vi "img test6.vi"() -> ()   [LabVIEW 2009]
uses:
  <vilib>/vision/NI_Vision_Development_Module.lvlib
panel:
  in  "start":i32
  out "Image 5":T1(plugin-control)
  out "Image 3":T1(plugin-control)
  in  "Range":cluster{"Lower value":sgl, "Upper value":sgl}={"Lower value"=30.0, "Upper value"=90.0} {"Upper value" format="%.2f"; "Lower value" format="%.2f"}
  out "Image 2":T1(plugin-control)
  in  "AVI Path":path=path "C:/Users/Kokum Weeratunga/Desktop/img processing/ChongWei vs LinDan (japan open 2010).avi"
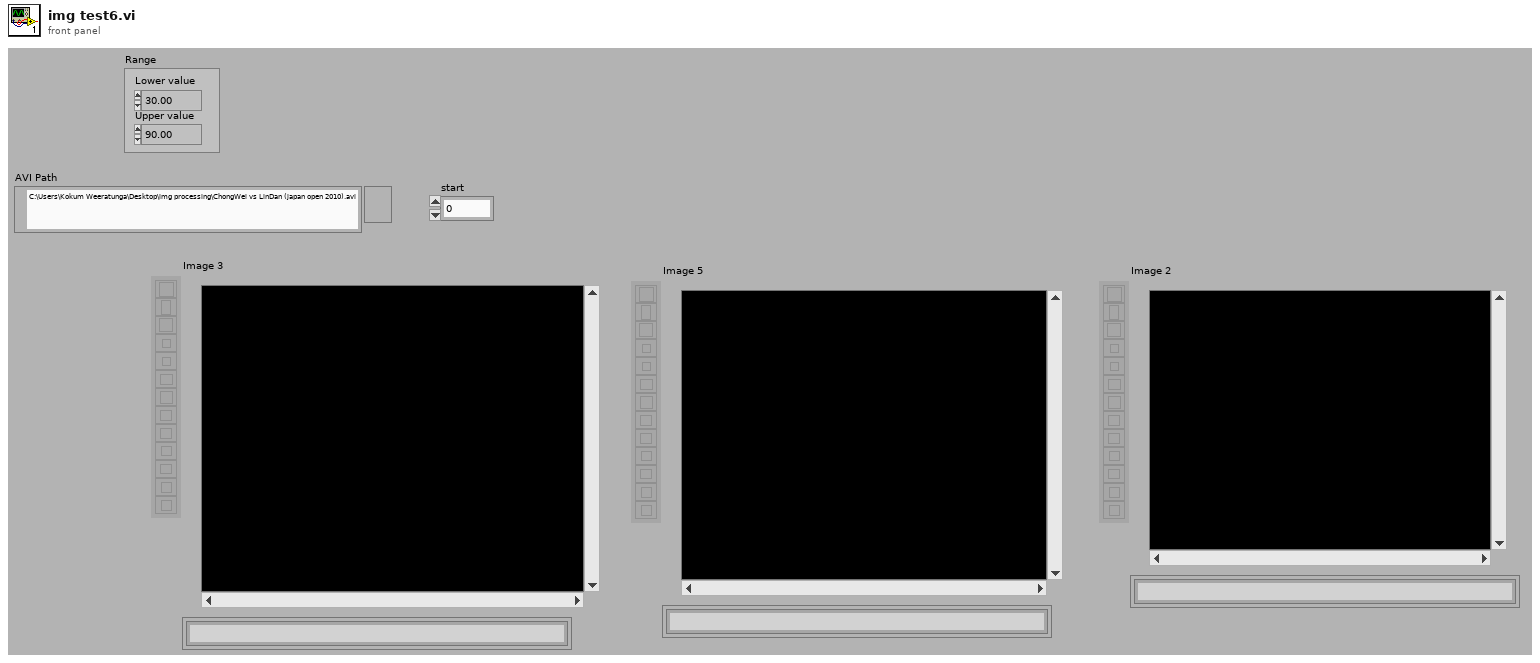
[diagram p1: front panel]
types:
  T1 = typedef "IMAQ Image.ctl" = refnum<image>
  T2 = typedef "Image Type" = u32
  T3 = typedef "AviRefnum.ctl" = refnum<k1>
  T4 = enum32{"AutoM", "Close", "Dilate", "Erode", "Gradient", "Gradient in", "Gradient out", "HitMiss", "Open", "PClose", "POpen", "Thick", "Thin"}
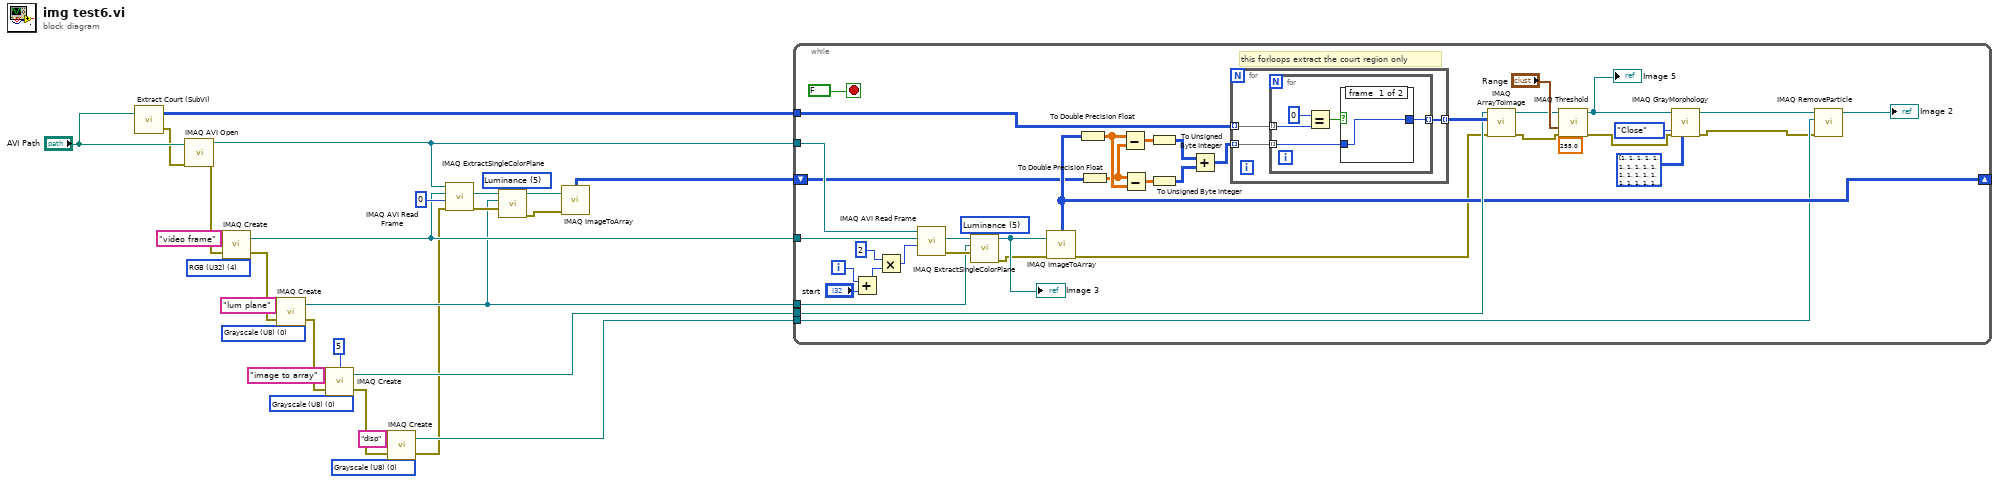
[diagram p0: block diagram]
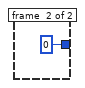
[diagram p2: hidden frame]
diagram:
  w10 = T2 0 items=["Grayscale (U8)", "Grayscale (I16)", "Grayscale (SGL)", "Complex (CSG)", "RGB (U32)", "HSL (U32)", "RGB (U64)", "Grayscale (U16)"] ("Image Type")
  w18 = 5 items=["Red", "Green", "Blue", "Hue", "Saturation", "Luminance", "Value", "Intensity"] ("Color Plane")
  w21 = T2 0 items=["Grayscale (U8)", "Grayscale (I16)", "Grayscale (SGL)", "Complex (CSG)", "RGB (U32)", "HSL (U32)", "RGB (U64)", "Grayscale (U16)"] ("Image Type")
  w25 = T2 0 items=["Grayscale (U8)", "Grayscale (I16)", "Grayscale (SGL)", "Complex (CSG)", "RGB (U32)", "HSL (U32)", "RGB (U64)", "Grayscale (U16)"] ("Image Type")
  w23 = T2 4 items=["Grayscale (U8)", "Grayscale (I16)", "Grayscale (SGL)", "Complex (CSG)", "RGB (U32)", "HSL (U32)", "RGB (U64)", "Grayscale (U16)"] ("Image Type")
  n1 = call "Extract Court (SubVI).vi"("AVI Path"="AVI Path") -> ("error out"=w28:errorcluster, "Court pixels out"=w26:u8[][])  [unwired: 1 in]
  n2 = call "IMAQ AVI Open"("error in (no error)"=w28, "AVI Path"="AVI Path") -> ("error out"=w5:errorcluster, "Avi Refnum"=w16:T3)  [unwired: 8 in]
  n3 = call "IMAQ Create"("Image Name"="video frame", "Image Type"=w23, "error in (no error)"=w5) -> ("New Image"=w14:T1, "error out"=w4:errorcluster)  [unwired: 2 in]
  n4 = call "IMAQ Create"("Image Name"="lum plane", "Image Type"=w25, "error in (no error)"=w4) -> ("New Image"=w13:T1, "error out"=w3:errorcluster)  [unwired: 2 in]
  n5 = call "IMAQ Create"("Border Size"=5, "Image Name"="image to array", "Image Type"=w21, "error in (no error)"=w3) -> ("New Image"=w20:T1, "error out"=w2:errorcluster)  [unwired: 1 in]
  n6 = call "IMAQ Create"("Image Name"="disp", "Image Type"=w10, "error in (no error)"=w2) -> ("New Image"=w8:T1, "error out"=w1:errorcluster)  [unwired: 2 in]
  n7 = call "IMAQ AVI Read Frame"("error in (no error)"=w1, "Frame Number"=u32 0, "Image"=w14, "Avi Refnum"=w16) -> ("error out"=w17:errorcluster, "Image Out"=w19:T1)  [unwired: 4 in, 2 out]
  n8 = call "IMAQ ExtractSingleColorPlane"("Color Plane"=w18, "error in (no error)"=w17, "Image Dst"=w13, "Image Src"=w19) -> ("error out"=w6:errorcluster, "Image Dst Out"=w11:T1)  [unwired: 6 in]
  n9 = call "IMAQ ImageToArray"("error in (no error)"=w6, "Image"=w11) -> ("Image Pixels (U8)"=w12:u8[][])  [unwired: 2 in, 4 out]
  n10 = while {
    tunnel: w16 -> [w66]
    tunnel: w14 -> [w65]
    tunnel: w26 -> [w64]
    tunnel: w13 -> [w55]
    tunnel: w20 -> [w56]
    shift-right: [w53] -> _
    shift-left: w12 -> [w52]
    tunnel: w8 -> [w36]
    i -> [w44]
    stop <- FALSE stop-if-true
    w67 = 5 items=["Red", "Green", "Blue", "Hue", "Saturation", "Luminance", "Value", "Intensity"] ("Color Plane")
    # "this forloops extract the court region only"
    n11 = Add(x=w44, y="start") -> (x+y=w43:i32)
    n12 = Multiply(x=2, y=w43) -> (x*y=w60:i32)
    n13 = call "IMAQ AVI Read Frame"("Frame Number"=w60, "Image"=w65, "Avi Refnum"=w66) -> ("error out"=w68:errorcluster, "Image Out"=w62:T1)  [unwired: 5 in, 2 out]
    n14 = call "IMAQ ExtractSingleColorPlane"("Color Plane"=w67, "error in (no error)"=w68, "Image Dst"=w55, "Image Src"=w62) -> ("error out"=w35:errorcluster, "Image Dst Out"=w54:T1)  [unwired: 6 in]
    "Image 3" <- w54
    n15 = call "IMAQ ImageToArray"("error in (no error)"=w35, "Image"=w54) -> ("error out"=w34:errorcluster, "Image Pixels (U8)"=w53:u8[][])  [unwired: 2 in, 3 out]
    n16 = To Double Precision Float(number=w53) -> (double precision float=w40:dbl[][])
    n17 = To Double Precision Float(number=w52) -> (double precision float=w39:dbl[][])
    n18 = Subtract(x=w40, y=w39) -> (x-y=w38:dbl[][])
    n19 = Subtract(x=w39, y=w40) -> (x-y=w37:dbl[][])
    n20 = To Unsigned Byte Integer(number=w38) -> (unsigned 8bit integer=w51:u8[][])
    n21 = To Unsigned Byte Integer(number=w37) -> (unsigned 8bit integer=w50:u8[][])
    n22 = Add(x=w51, y=w50) -> (x+y=w49:u8[][])
    n23 = for {
      tunnel: w64 -> [w71] mode=indexing
      tunnel: [w70] -> w61 mode=indexing
      tunnel: w49 -> [w69] mode=indexing
      n24 = for {
        tunnel: w71 -> [w76] mode=indexing
        tunnel: [w73] -> w70 mode=indexing
        tunnel: w69 -> [w72] mode=indexing
        n25 = Equal?(x=u8 0, y=w76) -> (x = y?=w74:bool)
        n26 = case shown="True" w74 {
          tunnel: [w77 u8 0 ("x")] -> w73
          tunnel: w72 -> [w77 _]
          frame #0 {
          }
          frame #1 {
          }
        }
      }
    }
    n27 = call "IMAQ ArrayToImage"("error in (no error)"=w34, "Image Pixels (U8)"=w61, "Image"=w56) -> ("error out"=w33:errorcluster, "Image Out"=w41:T1)  [unwired: 7 in]
    n28 = call "IMAQ Threshold"("Replace Value"=sgl 255.0, "error in (no error)"=w33, "Range"="Range", "Image Src"=w41) -> ("error out"=w32:errorcluster, "Image Dst Out"=w48:T1)  [unwired: 6 in]
    "Image 5" <- w48
    n29 = call "IMAQ GrayMorphology"("Structuring Element"=i32[][] [[1, 1, 1, 1, 1, 1, 1, 1, 1], [1, 1, 1, 1, 1, 1, 1, 1, 1], [1, 1, 1, 1, 1, 1, 1, 1, 1], [1, 1, 1, 1, 1, 1, 1, 1, 1], [1, 1, 1, 1, 1, 1, 1, 1, 1], [1, 1, 1, 1, 1, 1, 1, 1, 1], [1, 1, 1, 1, 1, 1, 1, 1, 1], [1, 1, 1, 1, 1, 1, 1, 1, 1], [1, 1, 1, 1, 1, 1, 1, 1, 1]], "error in (no error)"=w32, "Operation"=T4."Close", "Image Src"=w48) -> ("error out"=w30:errorcluster, "Image Dst Out"=w31:T1)  [unwired: 6 in]
    n30 = call "IMAQ RemoveParticle"("error in (no error)"=w30, "Image Dst"=w36, "Image Src"=w31) -> ("Image Dst Out"=→"Image 2":T1)  [unwired: 7 in, 1 out]
  }
